vi "Ke2000 Single Reading.vi"(8 "error in (no error)":errorcluster, 11 "VISA resource name":refnum<visa-resource-name>) -> (0 "error out":errorcluster, 1 "Units":string, 2 "Measurement":dbl, 3 "VISA resource name out":refnum<visa-resource-name>, 5 "uA":string)   [LabVIEW 2017]
panel:
  out "Channel":i32
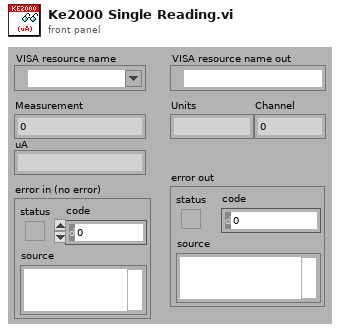
[diagram p1: front panel]
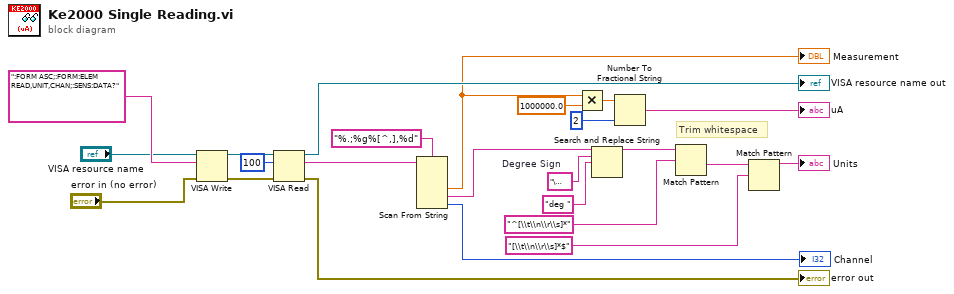
[diagram p0: block diagram]
diagram:
  w10 = "\u0013"  # Degree Sign
  # "Trim whitespace"
  n1 = VISA Write(VISA resource name="VISA resource name", write buffer=":FORM ASC;:FORM:ELEM READ,UNIT,CHAN;:SENS:DATA?", error in (no error)="error in (no error)") -> (VISA resource name out=w23:refnum<visa-resource-name>, error out=w22:errorcluster)  [unwired: 1 out]
  n2 = VISA Read(VISA resource name=w23, byte count=u32 100, error in (no error)=w22) -> (VISA resource name out=→"VISA resource name out":refnum<visa-resource-name>, read buffer=w8:string, error out=→"error out":errorcluster)  [unwired: 1 out]
  n3 = Scan From String(format string="%.;%g%[^,],%d", input string=w8) -> (output 1=w5:dbl, output 2=w11:string, output 3=→"Channel":i32)  [unwired: 5 in, 3 out]
  "Measurement" <- w5
  n4 = Multiply(x=w5, y=1000000.0) -> (x*y=w3:dbl)
  n5 = Search and Replace String(input string=w11, search string=w10, replace string="deg " ("replace string (\"\")")) -> (result string=w17:string)  [unwired: 5 in, 3 out]
  n6 = Number To Fractional String(number=w3, precision (6)=i16 2) -> (F-format string=→"uA":string)  [unwired: 2 in]
  n7 = Match Pattern(string=w17, regular expression="^[\\t\\n\\r\\s]*") -> (after substring=w14:string)  [unwired: 1 in, 3 out]
  n8 = Match Pattern(string=w14, regular expression="[\\t\\n\\r\\s]*$") -> (before substring=→"Units":string)  [unwired: 1 in, 3 out]
